vi "PKG_IMC_OpenUsePassword.vi"(7 "pwlen":i32, 9 "password":string, 10 "imcid":i32, 11 "netcardsel":i32) -> (1 "password out":string, 3 "function return":u32)   [LabVIEW 2011, in "IMC_Pkg4xxx.lvlib"]
doc: "PKG_IMC_OpenUsePassword (int netcardsel, int imcid, char *password, int pwlen);"
uses:
  IMC_Pkg4xxx.lvlib
  IMC_Pkg4xxx.dll
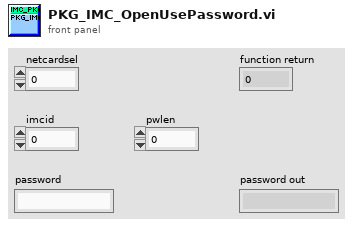
[diagram p1: front panel]
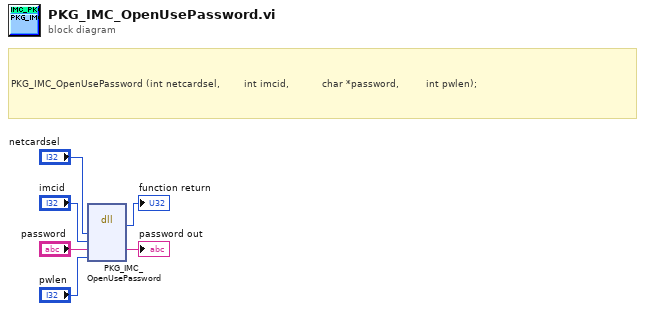
[diagram p0: block diagram]
diagram:
  # "PKG_IMC_OpenUsePassword (int netcardsel, \t\t\t\t\t\t\tint imcid,  \t\t\t\t\t\t\t\t\tchar *password,\t\t\t\t\t\t\t\t\tint pwlen);"
  n1 = dll-call lib="PTH1mabs F光盘刻录\niMC MotionIMCNet_V4.0IMCAppincLabviewIMC_PKG4xxxIMC_PKG4xxx\nIMC_Pkg4xxx.*" fn="PKG_IMC_OpenUsePassword"("netcardsel"="netcardsel", "imcid"="imcid", "password"="password", "pwlen"="pwlen") -> (→"function return":u32, "password"=→"password out":string)  [unwired: 6 in, 2 out]
